vi "SwerveLatchGoalAngle.vi"(1 "Raw Goal Angle":dbl format="%#_13g", 2 "In Deadband":bool) -> (0 "Latched Goal Angle":dbl)   [LabVIEW 2020]
doc: "Latches the goal azimuth angle when the driver releases the stick. This prevents the modules from slewing to a new orientation and jerking the robot or locking in an orientation that wold flip the robot."
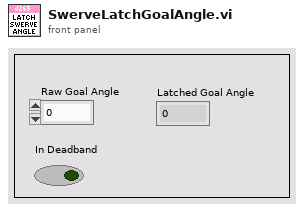
[diagram p1: front panel]
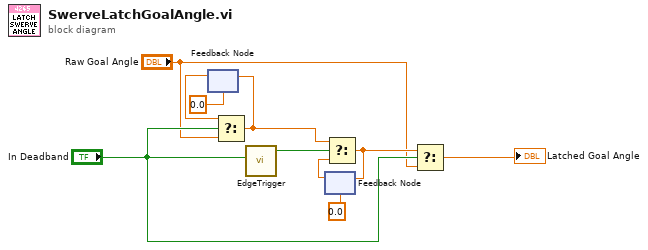
[diagram p0: block diagram]
diagram:
  n1 = feedback #1(0.0 ("Raw Goal Angle")) -> (w5:dbl)
  n2 = Select(t=w5, s="In Deadband", f="Raw Goal Angle") -> (s? t:f=w2:dbl)
  n3 = feedback-in #1(w2) -> ()
  n4 = call "EdgeTrigger.vi"("Input Signal"="In Deadband") -> ("Rising Edge Trigger"=w10:bool)  [unwired: 2 out]
  n5 = feedback #2(0.0) -> (w8:dbl)
  n6 = Select(t=w2, s=w10, f=w8) -> (s? t:f=w7:dbl)
  n7 = feedback-in #2(w7) -> ()
  n8 = Select(t=w7, s="In Deadband", f="Raw Goal Angle") -> (s? t:f=→"Latched Goal Angle":dbl)
